vi "acquire.vi"(5 "TDMS File Path":path, 7 "Logging Mode":i32(ring)=10231 items=["Off"=10231, "Log and Read"=15842], 8 "error in (no error)":errorcluster, 9 "Number of Samples":i32=100, 10 "Sample Rate":dbl=1000.0, 11 "Physical Channel":tag="Dev1/ai0") -> (0 "error out":errorcluster)   [LabVIEW 2019]
uses:
  <vilib>/Utility/error.llb/DialogType.ctl
  <vilib>/DAQmx/read.llb/DAQmx Read (Analog Wfm 1Chan NSamp).vi
  <vilib>/DAQmx/miscellaneous.llb/DAQmx Fill In Error Info.vi
  <vilib>/DAQmx/create/channels.llb/DAQmx Create Channel (AI-Voltage-Basic).vi
  <vilib>/DAQmx/configure/timing.llb/DAQmx Timing (Sample Clock).vi
  <vilib>/DAQmx/configure/task.llb/DAQmx Configure Logging (TDMS).vi
panel:
  out "Sinal":waveform(dbl)(graph)
  in  "Stop":bool
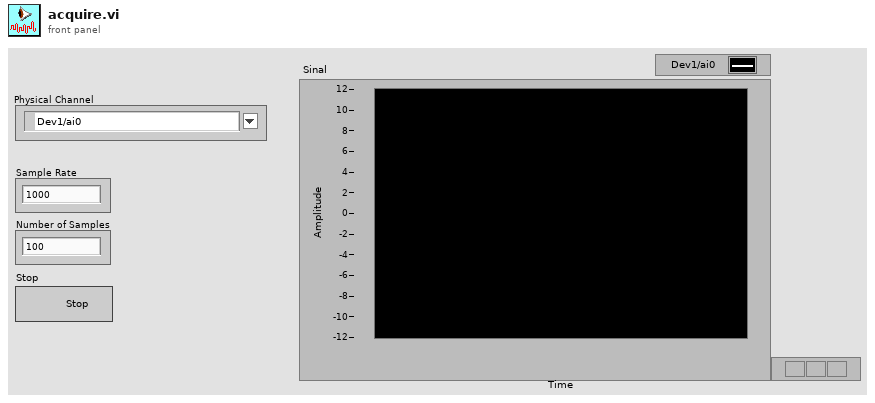
[diagram p1: front panel]
types:
  T1 = typedef "DialogType.ctl" = u16
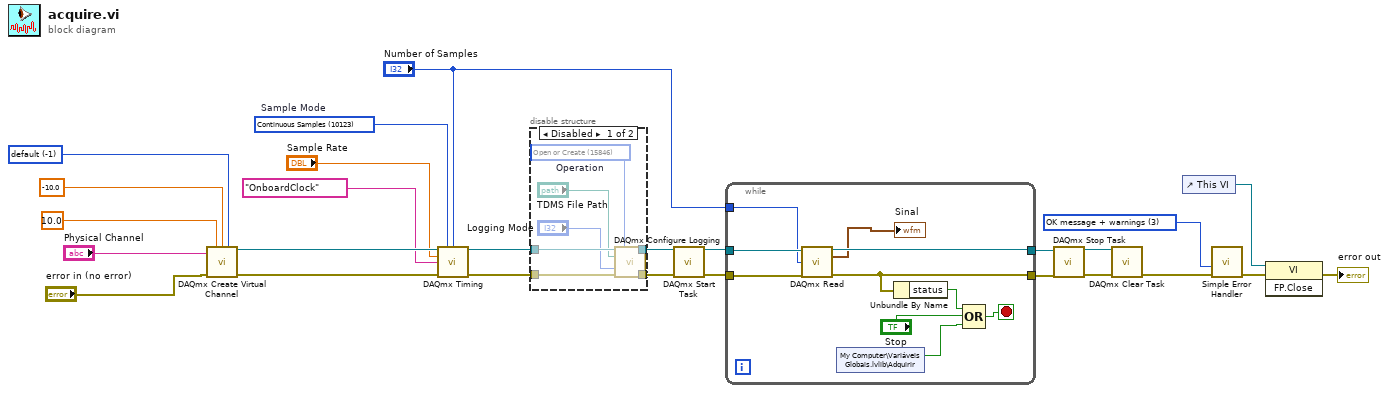
[diagram p0: block diagram]
diagram:
  w17 = -1 items=["default"=-1, "RSE"=10083, "NRSE"=10078, "Differential"=10106, "Pseudodifferential"=12529] ("Terminal Configuration")
  w7 = T1 3 items=["no dialog", "OK message", "continue or stop message", "OK message + warnings", "continue/stop + warnings"] ("type of dialog (OK msg:1)")
  w24 = 10123 items=["Finite Samples"=10178, "Continuous Samples"=10123, "Hardware Timed Single Point"=12522]  # Sample Mode
  n1 = call-poly <vilib>:"DAQmx Create Virtual Channel.vi"("maximum value"=10.0 ("Max Voltage"), "minimum value"=-10.0 ("Min Voltage"), "input terminal configuration"=w17, "physical channels"="Physical Channel", "error in"="error in (no error)") -> ("task out"=w22:refnum<k21>, "error out"=w23:errorcluster)  [unwired: 9 in]
  n2 = call-poly <vilib>:"DAQmx Timing.vi"("task/channels in"=w22, "sample mode"=w24, "samples per channel"="Number of Samples", "rate"="Sample Rate", "source"=tag "OnboardClock" ("Sample Clock Source"), "error in"=w23) -> ("task out"=w26:refnum<k21>, "error out"=w25:errorcluster)  [unwired: 8 in]
  n3 = disable-structure shown="Disabled" {
    disable-tunnel: w26 -> [w33 w35]
    disable-tunnel: w25 -> [w32 w34]
    disable-tunnel: [w28 w35] -> w6
    disable-tunnel: [w27 w34] -> w5
    frame Disabled {
      w31 = 15846 items=["Open"=10437, "Open or Create"=15846, "Create or Replace"=15847, "Create"=15848]  # Operation
      n4 = call-poly <vilib>:"DAQmx Configure Logging.vi"("task/channels in"=w33, "operation"=w31, "file path"="TDMS File Path", "logging mode"="Logging Mode", "error in"=w32) -> ("task out"=w28:refnum<k21>, "error out"=w27:errorcluster)  [unwired: 9 in]
    }
    frame Enabled {
    }
  }
  n5 = call <vilib>:"DAQmx Start Task.vi"("task/channels in"=w6, "error in"=w5) -> ("task out"=w21:refnum<k21>, "error out"=w20:errorcluster)  [unwired: 12 in]
  n6 = while {
    tunnel: w21 -> [w45]
    tunnel: w20 -> [w44]
    tunnel: [w43] -> w11
    tunnel: [w42] -> w10
    tunnel: "Number of Samples" -> [w39]
    stop <- w40 stop-if-true
    n7 = call-poly <vilib>:"DAQmx Read.vi"("task/channels in"=w45, "number of samples per channel"=w39, "error in"=w44) -> ("task out"=w43:refnum<k21>, "data"=→"Sinal":waveform(dbl), "error out"=w42:errorcluster)  [unwired: 10 in]
    n8 = shared-variable "My Computer\\Variáveis Globais.lvlib\\Adquirir"() -> (w36:bool)  [unwired: 1 in, 1 out]
    n9 = Unbundle By Name(w42) -> ("status"=w41:bool)
    n10 = Compound Arithmetic op=OR(w41, "Stop", w36) -> (w40:bool)
  }
  n11 = call <vilib>:"DAQmx Stop Task.vi"("task/channels in"=w11, "error in"=w10) -> ("task out"=w8:refnum<k21>, "error out"=w9:errorcluster)  [unwired: 12 in]
  n12 = call <vilib>:"DAQmx Clear Task.vi"("task in"=w8, "error in"=w9) -> ("error out"=w19:errorcluster)  [unwired: 13 in]
  n13 = control-ref of="This VI"() -> (w1:refnum<vi>)
  n14 = call <vilib>:"Simple Error Handler.vi"("type of dialog (OK msg:1)"=w7, "error in (no error)"=w19) -> ("error out"=w3:errorcluster)  [unwired: 3 in, 4 out]
  n15 = invoke class="VI" method="FP.Close"(reference=w1, error in=w3) -> (error out=→"error out":errorcluster)  [unwired: 1 in, 2 out]
